vi "RF CAR.vi"() -> ()   [LabVIEW 2018]
uses:
  <vilib>/MakerHub/LINX/Public/Peripherals/Digital/Digital Write 1 Chan.vi
  <vilib>/MakerHub/LINX/Public/Peripherals/Digital/Digital Write N Chans.vi
  <vilib>/MakerHub/LINX/Private/Local IO/LinxDigitalWrite.vi
  <vilib>/MakerHub/LINX/Public/Utilities/Check Channel.vi
  <vilib>/MakerHub/LINX/Public/Utilities/Open Serial.vi
  <vilib>/MakerHub/LINX/Private/Utilties/Generate Error.vi
  <vilib>/MakerHub/LINX/LMH-LINX.lvlib
panel:
  in  "stop":bool
  out "Loop Rate (Hz)":u32
  in  "Combo Box":string(combo)
  out "Forward":bool
  out "Left":bool
  out "Right":bool
  out "Reverse":bool
  out "STOP":bool
  in  "Serial Port":refnum<visa-resource-name>="N/A"
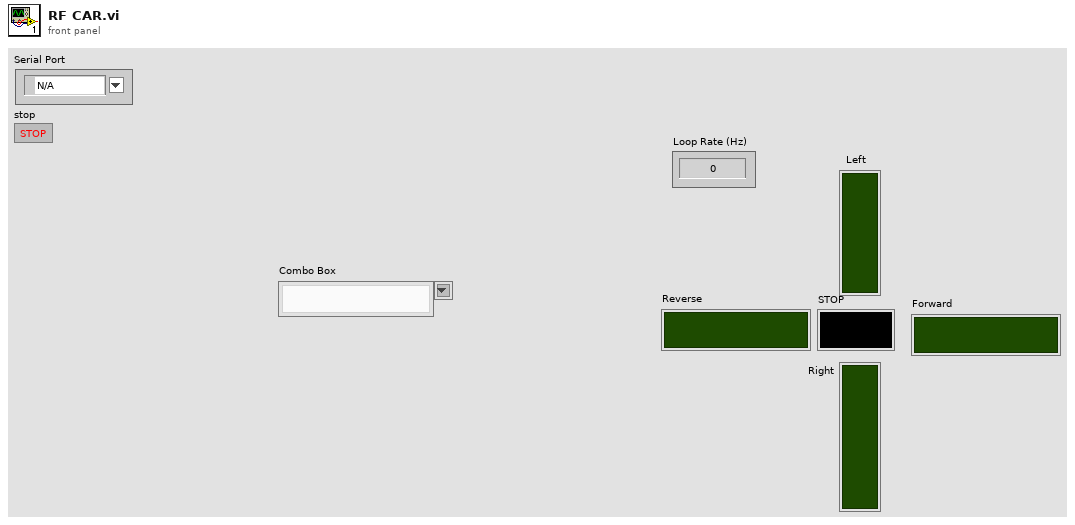
[diagram p1: front panel]
types:
  T1 = typedef "LMH-LINX.lvlib/LINX Ref.ctl" = cluster{"IO":T2, "Interface":T3, "LINX Device Config":T4}
  T2 = typedef "LMH-LINX.lvlib/Platform.ctl" = enum16{"Remote", "Local"}
  T3 = typedef "LMH-LINX.lvlib/Interface.ctl" = enum16{"Serial", "TCP"}
  T4 = typedef "LMH-LINX.lvlib/Device.lvlib/LINX Device Config.ctl" = cluster{"Interface":T3, "COM Port":refnum<visa-resource-name>, "TCP Configuration":T5, "Device Family":u8, "Device ID":u8, "Device Name":string, "TCP Ref":refnum<k5>, "Channels":T6}
  T5 = typedef "LMH-LINX.lvlib/Device.lvlib/TCP Config.ctl" = cluster{"IP Address":string, "Port":u16}
  T6 = typedef "LMH-LINX.lvlib/Channels.ctl" = cluster{"DI":u8[], "DO":u8[], "AI":u8[], "AO":u8[], "PWM":u8[], "QE":u8[], "UART":u8[], "I2C 2":u8[], "SPI":u8[], "CAN":u8[], "Servo":u8[], "AI Ref (V)":dbl, "AI Resolution (Bits)":u8, "AO Ref (V)":dbl, "AO Resolution (Bits)":u8}
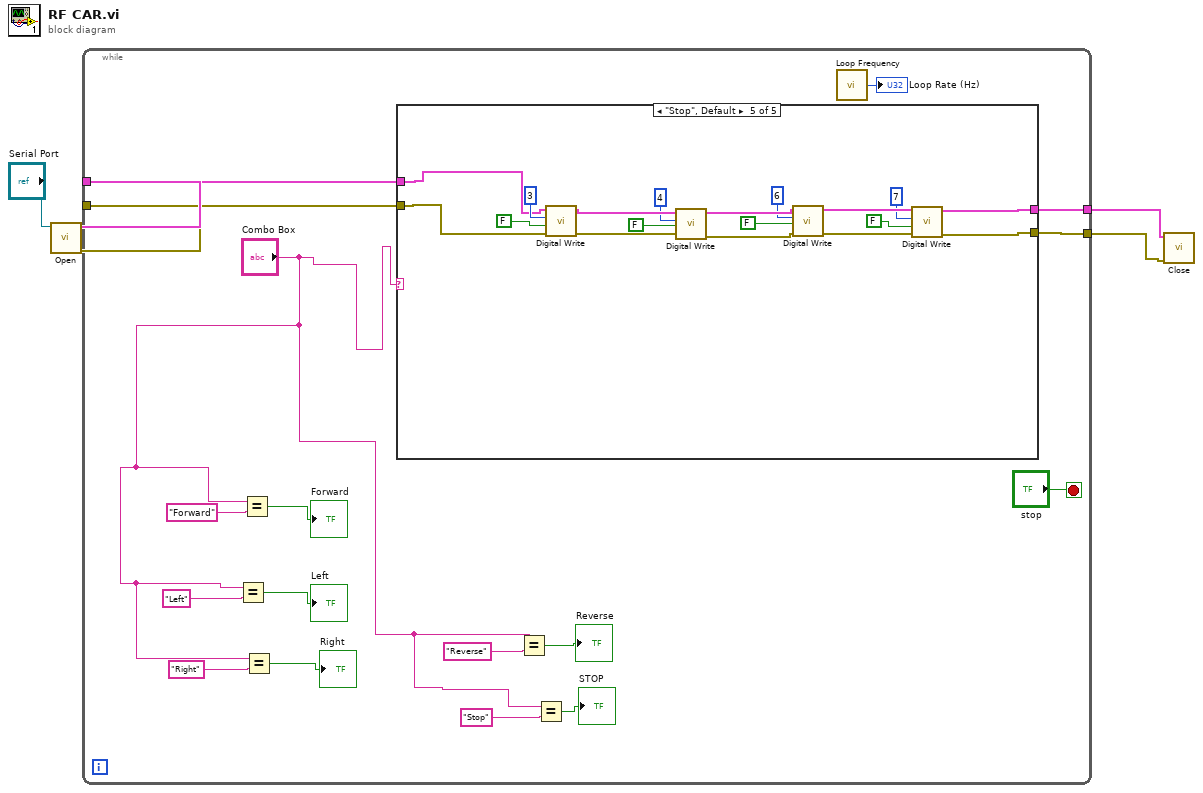
[diagram p0: block diagram]
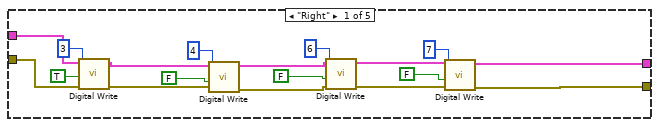
[diagram p2: hidden frame]
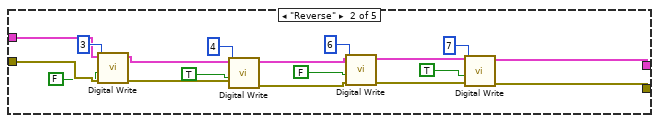
[diagram p3: hidden frame]
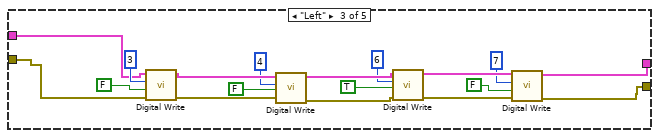
[diagram p4: hidden frame]
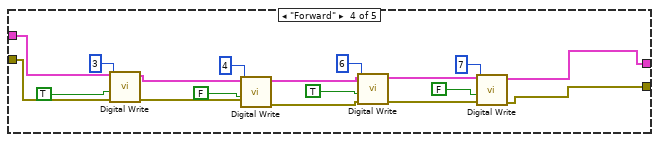
[diagram p5: hidden frame]
diagram:
  n1 = call-poly <vilib>:"Open.vi"("Serial Port"="Serial Port") -> ("Error Out"=w2:errorcluster, "LINX Resource"=w4:T1)  [unwired: 8 in, 1 out]
  n2 = while {
    tunnel: w4 -> [w22]
    tunnel: [w21] -> w3
    tunnel: w2 -> [w20]
    tunnel: [w19] -> w1
    stop <- "stop" stop-if-true
    n3 = Equal?(x="Combo Box", y="Left") -> (x = y?=→"Left":bool)
    n4 = Equal?(x="Combo Box", y="Forward") -> (x = y?=→"Forward":bool)
    n5 = Equal?(x="Combo Box", y="Right") -> (x = y?=→"Right":bool)
    n6 = case shown="\"Stop\", Default" "Combo Box" {
      tunnel: w22 -> [w40 w45 w61 w78 w96]
      tunnel: [w36 w42 w60 w81 w98] -> w21
      tunnel: w20 -> [w35 w44 w62 w77 w95]
      tunnel: [w31 w41 w59 w80 w97] -> w19
      frame "Right" {
        n7 = call-poly <vilib>:"Digital Write.vi"("Error In"=w35, "Output Value"=TRUE, "DO Channel"=u8 3, "LINX Resource"=w40) -> ("Error Out"=w34:errorcluster, "LINX Resource"=w39:T1)  [unwired: 6 in]
        n8 = call-poly <vilib>:"Digital Write.vi"("Error In"=w34, "Output Value"=FALSE ("RIGHT"), "DO Channel"=u8 4, "LINX Resource"=w39) -> ("Error Out"=w33:errorcluster, "LINX Resource"=w38:T1)  [unwired: 6 in]
        n9 = call-poly <vilib>:"Digital Write.vi"("Error In"=w33, "Output Value"=FALSE ("RIGHT"), "DO Channel"=u8 6, "LINX Resource"=w38) -> ("Error Out"=w32:errorcluster, "LINX Resource"=w37:T1)  [unwired: 6 in]
        n10 = call-poly <vilib>:"Digital Write.vi"("Error In"=w32, "Output Value"=FALSE ("RIGHT"), "DO Channel"=u8 7, "LINX Resource"=w37) -> ("Error Out"=w31:errorcluster, "LINX Resource"=w36:T1)  [unwired: 6 in]
      }
      frame "Reverse" {
        n11 = call-poly <vilib>:"Digital Write.vi"("Error In"=w44, "Output Value"=FALSE, "DO Channel"=u8 3, "LINX Resource"=w45) -> ("Error Out"=w55:errorcluster, "LINX Resource"=w58:T1)  [unwired: 6 in]
        n12 = call-poly <vilib>:"Digital Write.vi"("Error In"=w55, "Output Value"=TRUE ("RIGHT"), "DO Channel"=u8 4, "LINX Resource"=w58) -> ("Error Out"=w54:errorcluster, "LINX Resource"=w57:T1)  [unwired: 6 in]
        n13 = call-poly <vilib>:"Digital Write.vi"("Error In"=w54, "Output Value"=FALSE ("RIGHT"), "DO Channel"=u8 6, "LINX Resource"=w57) -> ("Error Out"=w53:errorcluster, "LINX Resource"=w56:T1)  [unwired: 6 in]
        n14 = call-poly <vilib>:"Digital Write.vi"("Error In"=w53, "Output Value"=TRUE ("RIGHT"), "DO Channel"=u8 7, "LINX Resource"=w56) -> ("Error Out"=w41:errorcluster, "LINX Resource"=w42:T1)  [unwired: 6 in]
      }
      frame "Left" {
        n15 = call-poly <vilib>:"Digital Write.vi"("Error In"=w62, "Output Value"=FALSE ("RIGHT"), "DO Channel"=u8 3, "LINX Resource"=w61) -> ("Error Out"=w74:errorcluster, "LINX Resource"=w71:T1)  [unwired: 6 in]
        n16 = call-poly <vilib>:"Digital Write.vi"("Error In"=w74, "Output Value"=FALSE ("RIGHT"), "DO Channel"=u8 4, "LINX Resource"=w71) -> ("Error Out"=w75:errorcluster, "LINX Resource"=w72:T1)  [unwired: 6 in]
        n17 = call-poly <vilib>:"Digital Write.vi"("Error In"=w75, "Output Value"=TRUE ("RIGHT"), "DO Channel"=u8 6, "LINX Resource"=w72) -> ("Error Out"=w76:errorcluster, "LINX Resource"=w73:T1)  [unwired: 6 in]
        n18 = call-poly <vilib>:"Digital Write.vi"("Error In"=w76, "Output Value"=FALSE ("RIGHT"), "DO Channel"=u8 7, "LINX Resource"=w73) -> ("Error Out"=w59:errorcluster, "LINX Resource"=w60:T1)  [unwired: 6 in]
      }
      frame "Forward" {
        n19 = call-poly <vilib>:"Digital Write.vi"("Error In"=w77, "Output Value"=TRUE ("RIGHT"), "DO Channel"=u8 3, "LINX Resource"=w78) -> ("Error Out"=w91:errorcluster, "LINX Resource"=w94:T1)  [unwired: 6 in]
        n20 = call-poly <vilib>:"Digital Write.vi"("Error In"=w91, "Output Value"=FALSE ("RIGHT"), "DO Channel"=u8 4, "LINX Resource"=w94) -> ("Error Out"=w90:errorcluster, "LINX Resource"=w93:T1)  [unwired: 6 in]
        n21 = call-poly <vilib>:"Digital Write.vi"("Error In"=w90, "Output Value"=TRUE ("RIGHT"), "DO Channel"=u8 6, "LINX Resource"=w93) -> ("Error Out"=w89:errorcluster, "LINX Resource"=w92:T1)  [unwired: 6 in]
        n22 = call-poly <vilib>:"Digital Write.vi"("Error In"=w89, "Output Value"=FALSE ("RIGHT"), "DO Channel"=u8 7, "LINX Resource"=w92) -> ("Error Out"=w80:errorcluster, "LINX Resource"=w81:T1)  [unwired: 6 in]
      }
      frame "Stop", Default {
        n23 = call-poly <vilib>:"Digital Write.vi"("Error In"=w95, "Output Value"=FALSE ("RIGHT"), "DO Channel"=u8 3, "LINX Resource"=w96) -> ("Error Out"=w110:errorcluster, "LINX Resource"=w107:T1)  [unwired: 6 in]
        n24 = call-poly <vilib>:"Digital Write.vi"("Error In"=w110, "Output Value"=FALSE ("RIGHT"), "DO Channel"=u8 4, "LINX Resource"=w107) -> ("Error Out"=w111:errorcluster, "LINX Resource"=w108:T1)  [unwired: 6 in]
        n25 = call-poly <vilib>:"Digital Write.vi"("Error In"=w111, "Output Value"=FALSE ("RIGHT"), "DO Channel"=u8 6, "LINX Resource"=w108) -> ("Error Out"=w112:errorcluster, "LINX Resource"=w109:T1)  [unwired: 6 in]
        n26 = call-poly <vilib>:"Digital Write.vi"("Error In"=w112, "Output Value"=FALSE ("RIGHT"), "DO Channel"=u8 7, "LINX Resource"=w109) -> ("Error Out"=w97:errorcluster, "LINX Resource"=w98:T1)  [unwired: 6 in]
      }
    }
    n27 = Equal?(x="Combo Box", y="Reverse") -> (x = y?=→"Reverse":bool)
    n28 = Equal?(x="Combo Box", y="Stop") -> (x = y?=→"STOP":bool)
    n29 = call <vilib>:"Loop Frequency.vi"() -> ("Loop Rate (Hz)"=→"Loop Rate (Hz)":u32)
  }
  n30 = call <vilib>:"Close.vi"("Error In"=w1, "LINX Resource"=w3) -> ()  [unwired: 9 in, 1 out]
